vi "SCLN_InitGlobals.vi"   [LabVIEW 2015]
uses:
  SCLN_RW_Select.ctl
  SCLN_INT32_Select.ctl
types:
  T1 = typedef "SCLN_INT32_Select.ctl" = enum16{"Max_Servers", "Max_Clients", "Total_Servers", "Total_Clients"}
  T2 = typedef "SCLN_RW_Select.ctl" = enum16{"Read", "Write"}
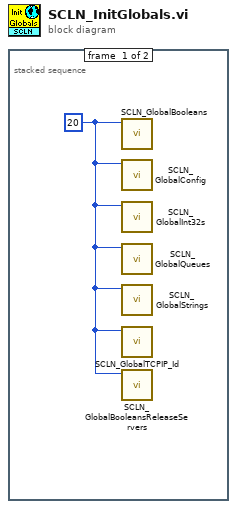
[diagram p0: block diagram]
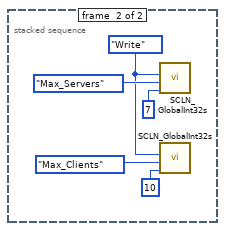
[diagram p2: hidden frame]
diagram:
  n1 = stacked-sequence {
    frame #0 {
      w1 = 20
      n2 = call "SCLN_GlobalBooleans.vi"("Number of Elements"=w1) -> ()  [unwired: 3 in, 2 out]
      n3 = call "SCLN_GlobalConfig.vi"("Number of Elements"=w1) -> ()  [unwired: 3 in, 2 out]
      n4 = call "SCLN_GlobalInt32s.vi"("Number of Elements"=w1) -> ()  [unwired: 3 in, 2 out]
      n5 = call "SCLN_GlobalQueues.vi"("Number of Elements"=w1) -> ()  [unwired: 7 in, 2 out]
      n6 = call "SCLN_GlobalStrings.vi"("Number of Elements"=w1) -> ()  [unwired: 3 in, 2 out]
      n7 = call "SCLN_GlobalTCPIP_Id.vi"("Number of elements"=w1) -> ()  [unwired: 3 in, 2 out]
      n8 = call "SCLN_GlobalBooleansReleaseServers.vi"("Number of Elements"=w1) -> ()  [unwired: 3 in, 2 out]
    }
    frame #1 {
      w4 = SCLN_RW_Select."Write" ("GBL_RW")
      n9 = call "SCLN_GlobalInt32s.vi"("Write Value"=7, "Element"=SCLN_INT32_Select."Max_Servers" ("GBL_INT32"), "Operation"=w4) -> ()  [unwired: 1 in, 2 out]
      n10 = call "SCLN_GlobalInt32s.vi"("Write Value"=10, "Element"=SCLN_INT32_Select."Max_Clients" ("GBL_INT32"), "Operation"=w4) -> ()  [unwired: 1 in, 2 out]
    }
  }
